vi "Get Routing Channel Initial State.vi"(8 "error in":errorcluster, 11 "routing channel in":T1 format="%.0x") -> (0 "error out":errorcluster, 2 "initial state":string, 3 "routing channel out":T1=18446744073709551615 format="%.0x")   [LabVIEW 2020, in "Routing and Faulting Scripting.lvlib"]
doc: "Returns the name of the initial state of the routing channel."
uses:
  Routing and Faulting Scripting.lvlib
  <vilib>/NI VeriStand/Custom Device API/Custom Device Item Ref.ctl
  Shared/Convert State Value to Integer.vi
  <vilib>/Utility/error.llb/Error Cluster From Error Code.vi
  <vilib>/NI VeriStand/Custom Device API/Custom Device API.lvlib
  Dependencies.llb/Routing and Faulting Shared.lvlib
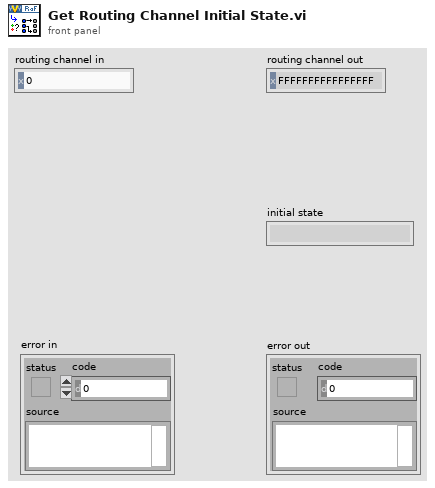
[diagram p1: front panel]
types:
  T1 = typedef "Custom Device API.lvlib/Custom Device Item Ref.ctl" = u64
  T2 = typedef "Custom Device API.lvlib/Custom Device Channel.ctl" = cluster{"Type":T3, "Units":string, "Default Value":dbl, "Faultable":bool, "Scalable":bool}
  T3 = typedef "Custom Device API.lvlib/Custom Device Channel Type.ctl" = enum16{"Input", "Output"}
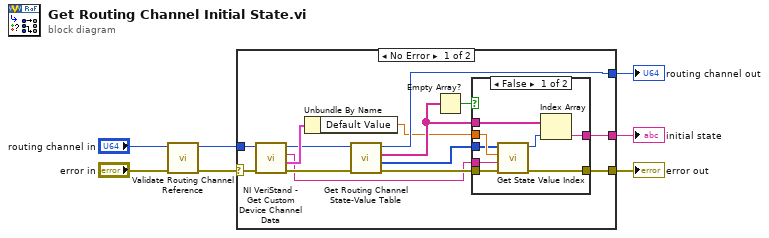
[diagram p0: block diagram]
diagram:
  n1 = call "Validate Routing Channel Reference.vi"("error in"="error in", "routing channel in"="routing channel in") -> ("error out"=w3:errorcluster, "routing channel out"=w1:T1)  [unwired: 8 in]
  n2 = case shown="No Error" w3 {
    selector: w3 -> [w19 w32]
    tunnel: [w13 w32] -> w5
    tunnel: w1 -> [w21 w31]
    tunnel: [w17 w31] -> w6
    tunnel: [w11 _] -> w4
    frame No Error {
      n3 = call <vilib>:"NI VeriStand - Get Custom Device Channel Data.vi"("error in (no error)"=w19, "Channel Ref in"=w21) -> ("error out"=w16:errorcluster, "Channel"=w20:T2, "Channel Name"=w10:string, "Channel Ref out"=w18:T1)  [unwired: 4 in, 2 out]
      n4 = Unbundle By Name(w20) -> ("Default Value"=w9:dbl)
      n5 = call "Get Routing Channel State-Value Table.vi"("error in"=w16, "routing channel in"=w18) -> ("error out"=w15:errorcluster, "state values"=w8:i32[], "state names"=w12:string[], "routing channel out"=w17:T1)  [unwired: 6 in]
      n6 = Empty Array?(array=w12) -> (empty?=w14:bool)
      n7 = case shown="False" w14 {
        tunnel: w15 -> [w29 w30]
        tunnel: w9 -> [w28 _]
        tunnel: w8 -> [w27 _]
        tunnel: [w26 w30] -> w13
        tunnel: w12 -> [w25 _]
        tunnel: [w23 _] -> w11
        tunnel: w10 -> [w22 _]
        frame False {
          n8 = call "Get State Value Index.vi"("error in (no error)"=w29, "Channel Name"=w22, "State Value"=w28, "State Value Array"=w27) -> ("error out"=w26:errorcluster, "index of element"=w24:i32)  [unwired: 6 in]
          n9 = Index Array(array=w25, index=w24) -> (element=w23:string)
        }
        frame True {
        }
      }
    }
    frame Error {
    }
  }
  "routing channel out" <- w6
  "error out" <- w5
  "initial state" <- w4
